vi "Call Count.vi"(8 "error in (no error)":errorcluster, 11 "LabSpy in":refnum<class "LabSpy.lvclass">) -> (0 "error out":errorcluster, 2 "Call Count":i32, 3 "LabSpy out":refnum<class "LabSpy.lvclass">)   [LabVIEW 2013, in "LabSpy.lvclass"]
doc: "Reads the number of times the spy has been called."
uses:
  LabSpy.lvclass
  LabSpy.lvclass/LabSpy.ctl
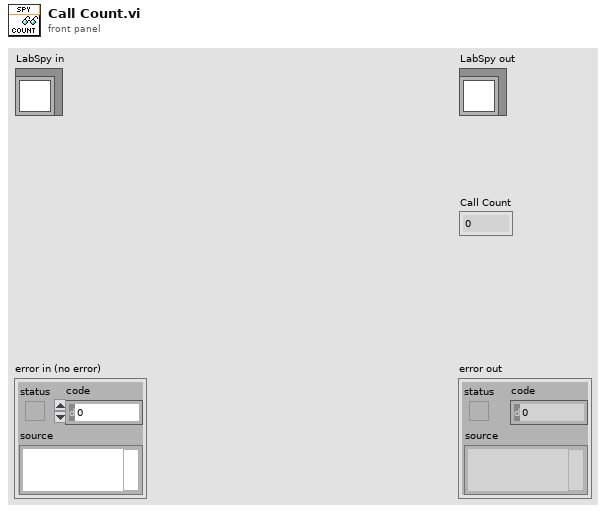
[diagram p1: front panel]
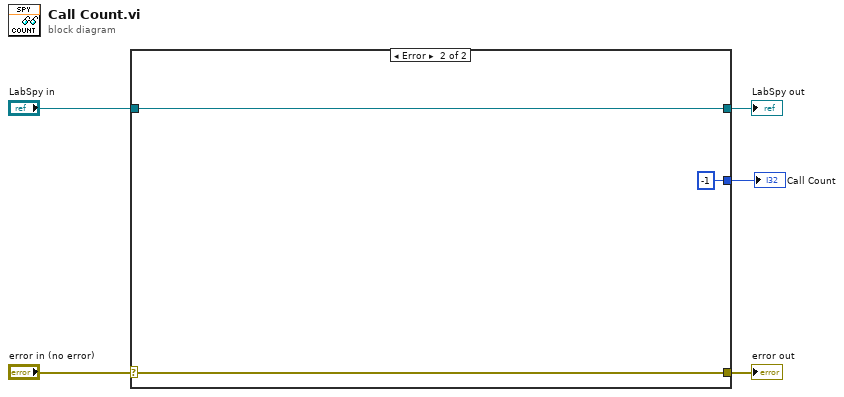
[diagram p0: block diagram]
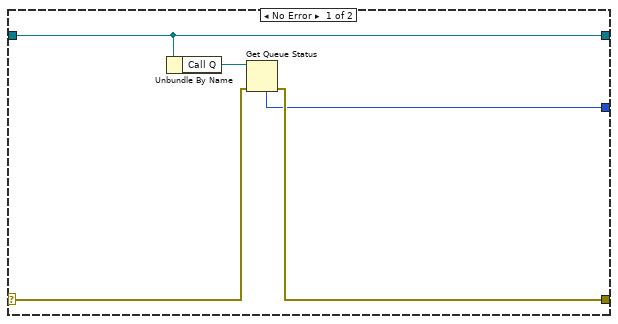
[diagram p2: hidden frame]
diagram:
  n1 = case shown="Error" "error in (no error)" {
    selector: "error in (no error)" -> [w8 w13]
    tunnel: [w7 w13] -> w4
    tunnel: [w10 w12] -> w2
    tunnel: "LabSpy in" -> [w10 w12]
    tunnel: [w6 -1 ("# elements in queue")] -> w1
    frame No Error {
      n2 = Unbundle By Name(w10) -> ("Call Q"=w9:refnum<queue>)
      n3 = Get Queue Status(queue=w9, error in (no error)=w8) -> (error out=w7:errorcluster, # elements in queue=w6:i32)  [unwired: 1 in, 6 out]
    }
    frame Error {
    }
  }
  "error out" <- w4
  "LabSpy out" <- w2
  "Call Count" <- w1
